vi "子VI-深度学习自动检测结果分析.vi"(0 "计入缺陷的Z值阈值":i32 caption="值", 1 "判定为筋条的长宽比阈值":i32, 2 "临界Z值":i32, 3 "缺陷灰度阈值":dbl caption="值", 4 "临界面积百分比值":dbl, 5 "计入缺陷的面积阈值":i32, 6 "预测图片保存路径":path) -> (16 "全部检测结果":string[][](table), 19 "Threshold Image":T2(plugin-control))   [LabVIEW 2018]
uses:
  <vilib>/vision/NI_Vision_Development_Module.lvlib
panel:
  in  "Tab Control":T1
  out "?":T2(plugin-control)
  out "分层缺陷个数":i32
  out "合格？ 弥散类":string="fencengThreshold"
  out "合格？分层类":string="fencengThreshold"
  out "面积 (pixels)":i32
  in  "格式字符串 2":string="%f"
  in  "分隔符（'\\'代码显示）":string="\t"
  # "所选区域信息"
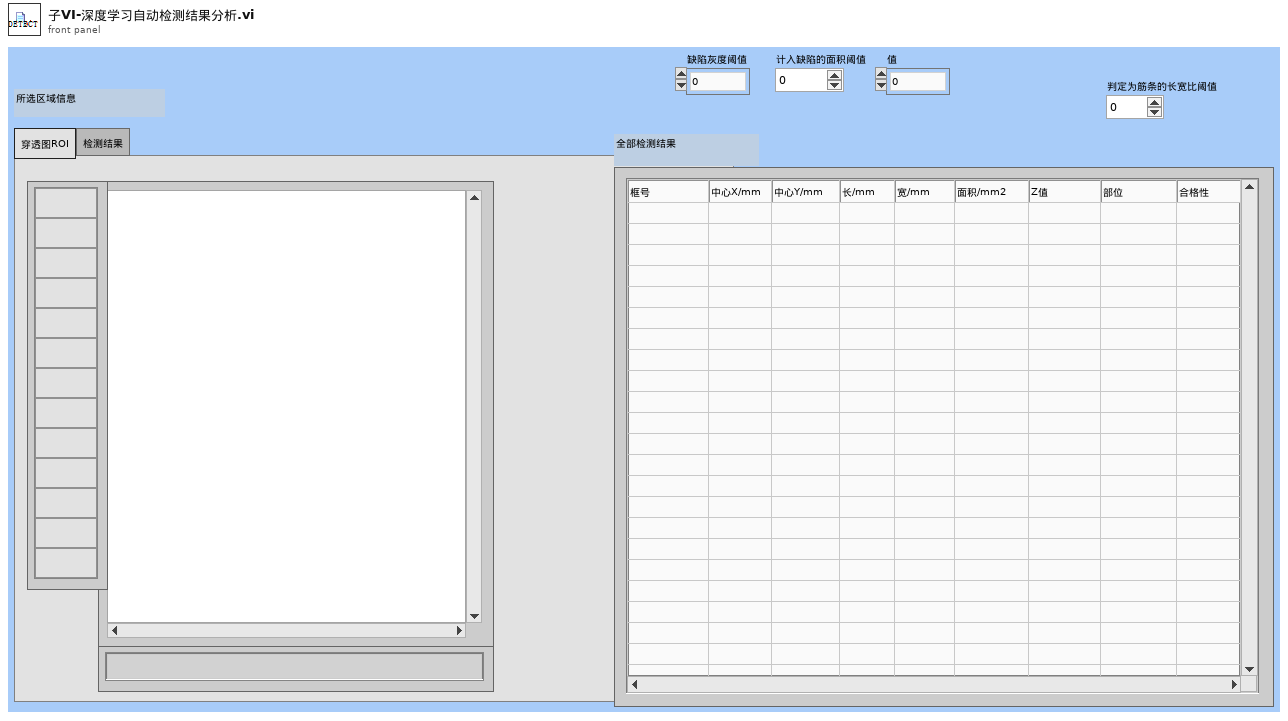
[diagram p1: front panel]
types:
  T1 = typedef "控件2.ctl" = enum32{"穿透图ROI", "检测结果"}
  T2 = typedef "IMAQ Image.ctl" = refnum<image>
  T3 = typedef "Image Type" = u32
  T4 = cluster{"histogram":u32[], "Minimal Value":sgl, "Maximal Value":sgl, "Starting Value":sgl, "Interval Width":sgl, "Mean Value":sgl, "Standard  Variation":sgl, "Area (pixels)":i32}
  T5 = cluster{"Area":dbl, "Number of Holes":dbl, "Bounding Rect":cluster{"Left":dbl, "Top":dbl, "Right":dbl, "Bottom":dbl}, "Center of Mass":cluster{"X":dbl, "Y":dbl}, "Orientation":dbl, "Dimensions":cluster{"Width":dbl, "Height":dbl}}[]
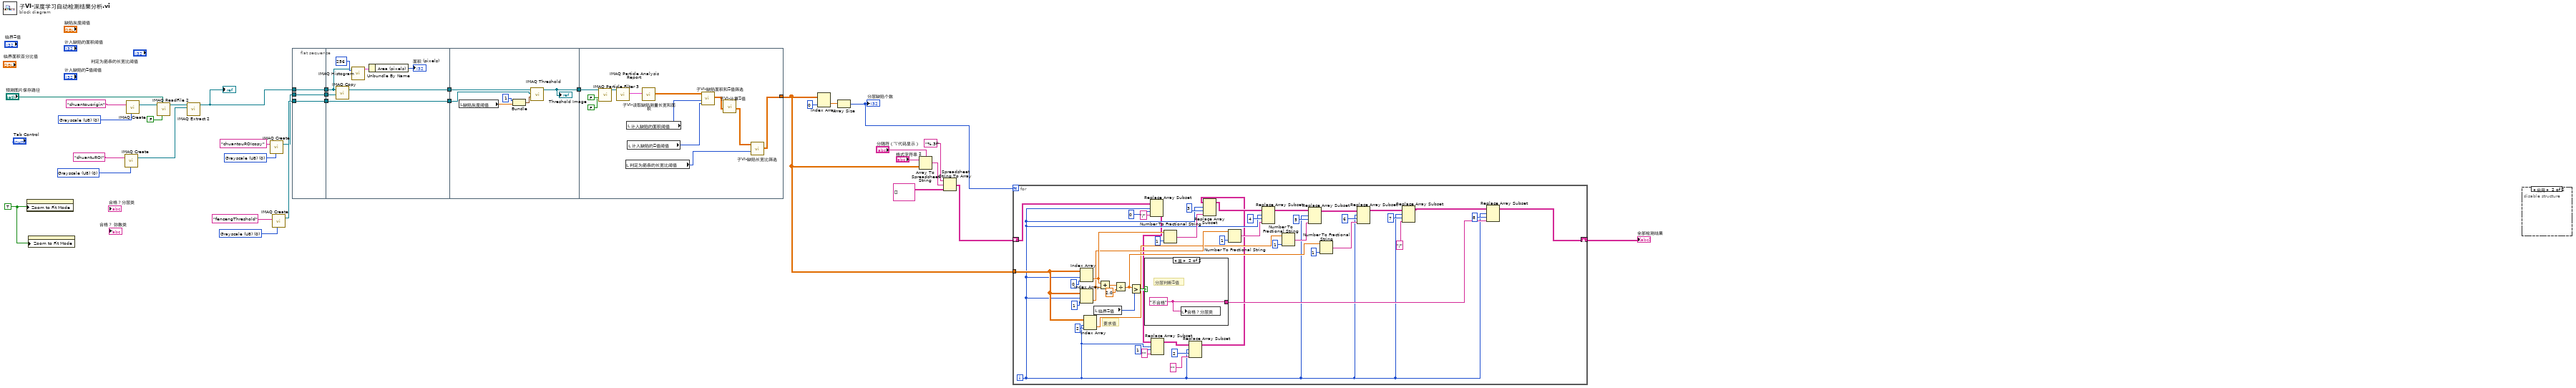
[diagram p0: block diagram]
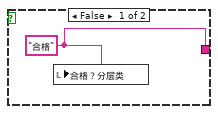
[diagram p2: hidden frame]
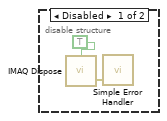
[diagram p3: hidden frame]
diagram:
  w2 = T3 0 items=["Grayscale (U8)", "Grayscale (I16)", "Grayscale (SGL)", "Complex (CSG)", "RGB (U32)", "HSL (U32)", "RGB (U64)", "Grayscale (U16)"] ("Image Type")
  w7 = TRUE ("Zoom to Fit Mode")
  w24 = T3 0 items=["Grayscale (U8)", "Grayscale (I16)", "Grayscale (SGL)", "Complex (CSG)", "RGB (U32)", "HSL (U32)", "RGB (U64)", "Grayscale (U16)"] ("Image Type")
  w27 = T3 0 items=["Grayscale (U8)", "Grayscale (I16)", "Grayscale (SGL)", "Complex (CSG)", "RGB (U32)", "HSL (U32)", "RGB (U64)", "Grayscale (U16)"] ("Image Type")
  w33 = T3 0 items=["Grayscale (U8)", "Grayscale (I16)", "Grayscale (SGL)", "Complex (CSG)", "RGB (U32)", "HSL (U32)", "RGB (U64)", "Grayscale (U16)"] ("Image Type")
  n1 = property class="ImageControl"("Zoom to Fit Mode"=w7) -> ()  [unwired: 2 in, 2 out]
  n2 = property class="ImageControl"("Zoom to Fit Mode"=w7) -> ()  [unwired: 2 in, 2 out]
  n3 = call "IMAQ Create"("Image Name"="chuantuROI", "Image Type"=w27) -> ("New Image"=w26:T2)  [unwired: 3 in, 1 out]
  n4 = call "IMAQ Create"("Image Name"="chuantouorigin", "Image Type"=w33) -> ("New Image"=w29:T2)  [unwired: 3 in, 1 out]
  n5 = call "IMAQ ReadFile 2"("Use File Path Image Type"=FALSE, "File Path"="预测图片保存路径", "Image"=w29) -> ("Image Out"=w30:T2)  [unwired: 4 in, 4 out]
  n6 = call "IMAQ Extract 2"("Image Dst"=w26, "Image Src"=w30) -> ("Image Dst Out"=w9:T2)  [unwired: 8 in, 1 out]
  "?" <- w9
  n7 = call "IMAQ Create"("Image Name"="chuantouROIcopy", "Image Type"=w2) -> ("New Image"=w5:T2)  [unwired: 3 in, 1 out]
  n8 = call "IMAQ Create"("Image Name"="fencengThreshold", "Image Type"=w24) -> ("New Image"=w20:T2)  [unwired: 3 in, 1 out]
  n9 = flat-sequence {
    tunnel: w9 -> [w36]
    tunnel: [w37] -> w21
    tunnel: w20 -> [w37]
    tunnel: [w36] -> w8
    tunnel: w5 -> [w35]
    tunnel: [w35] -> w4
    tunnel: [w44] -> w19
    tunnel: w21 -> [w44]
    tunnel: w8 -> [w40]
    tunnel: [w39] -> w6
    tunnel: w4 -> [w38]
    tunnel: w19 -> [w50]
    tunnel: [w49] -> w18
    tunnel: w6 -> [w48]
    tunnel: [w55] -> w11
    tunnel: w18 -> [w60]
    frame #0 {
    }
    frame #1 {
      n10 = call "IMAQ Copy"("Image Dst"=w38, "Image Src"=w40) -> ("Image Dst Out"=w39:T2)  [unwired: 4 in, 1 out]
      n11 = call "IMAQ Histogram"("Number of Classes"=256, "Image"=w40) -> ("Histogram Report"=w42:T4)  [unwired: 8 in, 1 out]
      n12 = Unbundle By Name(w42) -> ("Area (pixels)"=→"面积 (pixels)":i32)
    }
    frame #2 {
      n13 = local read "缺陷灰度阈值"() -> (w46:dbl)
      n14 = Bundle(1, "缺陷灰度阈值"=w46) -> (w45:cluster{i32, "缺陷灰度阈值":dbl})  [unwired: 1 in]
      n15 = call "IMAQ Threshold"("Range"=w45, "Image Dst"=w50, "Image Src"=w48) -> ("Image Dst Out"=w49:T2)  [unwired: 3 in, 5 out]
      "Threshold Image" <- w49
    }
    frame #3 {
      n16 = call "IMAQ Particle Filter 3"("Image Src"=w60, "Keep/Remove Particles (F)"=FALSE, "Reject Border? (F)"=FALSE) -> ("Image Dst Out"=w59:T2)  [unwired: 10 in, 2 out]
      n17 = call "IMAQ Particle Analysis Report"("Image"=w59) -> ("Particle Reports (Pixels)"=w58:T5)  [unwired: 5 in, 5 out]
      n18 = local read "判定为筋条的长宽比阈值"() -> (w54:i32)
      n19 = local read "计入缺陷的面积阈值"() -> (w56:i32)
      n20 = local read "计入缺陷的Z值阈值"() -> (w52:i32)
      n21 = call "子VI-读取缺陷测量长宽和面积.vi"("Particle Reports (Pixels)"=w58) -> ("测量结果"=w57:dbl[][])  [unwired: 10 in]
      n22 = call "子VI-缺陷面积和Z值筛选.vi"("计入缺陷的Z值阈值"=w52, "计入分层缺陷的面积阈值"=w56, "分层测量结果"=w57) -> ("初始化的数组"=w53:dbl[][])  [unwired: 7 in, 1 out]
      n23 = call "子VI-计算Z值.vi"("分层测量结果"=w53) -> ("初始化的数组"=w51:dbl[][])  [unwired: 9 in]
      n24 = call "子VI-缺陷长宽比筛选.vi"("判定为筋条的长宽比阈值"=w54, "分层测量结果"=w51) -> ("初始化的数组"=w55:dbl[][])  [unwired: 9 in]
    }
  }
  n25 = Index Array(array=w11, index (col)=0 ("禁用的索引 (列)")) -> (element=w23:dbl[])  [unwired: 1 in]
  n26 = Array Size(array=w23) -> (size(s)=w17:i32)
  "分层缺陷个数" <- w17
  n27 = Array To Spreadsheet String(delimiter (Tab)="分隔符（'\\'代码显示）", array=w11, 3:"格式字符串 2") -> (spreadsheet string=w14:string)
  n28 = Spreadsheet String To Array(format string="%.3f", spreadsheet string=w14, array type (2D Dbl)=string[][] [] ("Array")) -> (array=w10:string[][])  [unwired: 1 in]
  n29 = for {
    N: w17 -> [_]
    tunnel: w11 -> [w79]
    shift-right: [w86] -> w1
    shift-left: w10 -> [w94]
    i -> [w71]
    # "要求值"
    n30 = Index Array(array=w79, index (row)=w71, index (col)=0 ("禁用的索引 (列)")) -> (element=w85:dbl)
    n31 = Index Array(array=w79, index (row)=w71, index (col)=1 ("禁用的索引 (列)")) -> (element=w84:dbl)
    n32 = Index Array(array=w79, index (row)=w71, index (col)=2 ("禁用的索引 (列)")) -> (element=w77:dbl)
    n33 = local read "临界Z值"() -> (w105:i32)
    n34 = Add(x=w85, y=w84) -> (x+y=w106:dbl)
    n35 = Divide(x=w106, y=2.0) -> (x/y=w82:dbl)
    n36 = Greater?(x=w82, y=w105) -> (0:w107:bool)
    n37 = case shown="真" w107 {
      tunnel: [w108 w109] -> w81
      frame False {
        w108 = "合格" ("合格？")
        n38 = local write "合格？分层类"(w108) -> ()
      }
      frame True {
        w109 = "不合格" ("合格？")
        # "分层判断Z值"
        n39 = local write "合格？分层类"(w109) -> ()
      }
    }
    n40 = Replace Array Subset(array=w94, new element="/" ("新元素/子数组"), index (row)=w71, index (col)=0 ("索引 (列)")) -> (w69:string[][])
    n41 = Replace Array Subset(array=w69, new element="" ("新元素/子数组"), index (row)=w71, index (col)=1 ("索引 (列)")) -> (w74:string[][])
    n42 = Number To Fractional String(number=w85, precision (6)=i16 1 ("精度(6)")) -> (F-format string=w93:string)  [unwired: 2 in]
    n43 = Replace Array Subset(array=w74, new element="" ("新元素/子数组"), index (row)=w71, index (col)=2 ("索引 (列)")) -> (w68:string[][])
    n44 = Replace Array Subset(array=w68, new element=w93, index (row)=w71, index (col)=3 ("索引 (列)")) -> (w91:string[][])
    n45 = Number To Fractional String(number=w84, precision (6)=i16 1 ("精度(6)")) -> (F-format string=w92:string)  [unwired: 2 in]
    n46 = Replace Array Subset(array=w91, new element=w92, index (row)=w71, index (col)=4 ("索引 (列)")) -> (w90:string[][])
    n47 = Number To Fractional String(number=w77, precision (6)=i16 1 ("精度(6)")) -> (F-format string=w89:string)  [unwired: 2 in]
    n48 = Replace Array Subset(array=w90, new element=w89, index (row)=w71, index (col)=5 ("索引 (列)")) -> (w88:string[][])
    n49 = Number To Fractional String(number=w82, precision (6)=i16 1 ("精度(6)")) -> (F-format string=w83:string)  [unwired: 2 in]
    n50 = Replace Array Subset(array=w88, new element=w83, index (row)=w71, index (col)=6 ("索引 (列)")) -> (w87:string[][])
    n51 = Replace Array Subset(array=w87, new element="/" ("新元素/子数组"), index (row)=w71, index (col)=7 ("索引 (列)")) -> (w63:string[][])
    n52 = Replace Array Subset(array=w63, new element=w81, index (row)=w71, index (col)=8 ("索引 (列)")) -> (w86:string[][])
  }
  "全部检测结果" <- w1
  n53 = disable-structure shown="启用" {
    frame Disabled {
      n54 = call "IMAQ Dispose"("All Images? (No)"=TRUE) -> ("error out"=w111:errorcluster)  [unwired: 5 in]
      n55 = call <vilib>:"Simple Error Handler.vi"("error in (no error)"=w111) -> ()  [unwired: 4 in, 5 out]
    }
    frame Enabled {
    }
  }
